vi "CleanUp.vi"(0 "object in":refnum<class "Valve.lvclass">, 5 "error in (no error)":errorcluster) -> (14 "object out":refnum<class "Valve.lvclass">, 19 "error out":errorcluster)   [LabVIEW 2019, in "Valve.lvclass"]
uses:
  Valve.lvclass
  Valve.lvclass/Valve.ctl
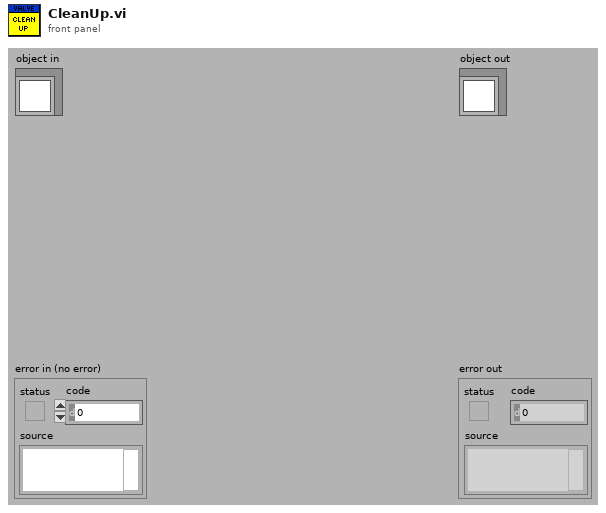
[diagram p1: front panel]
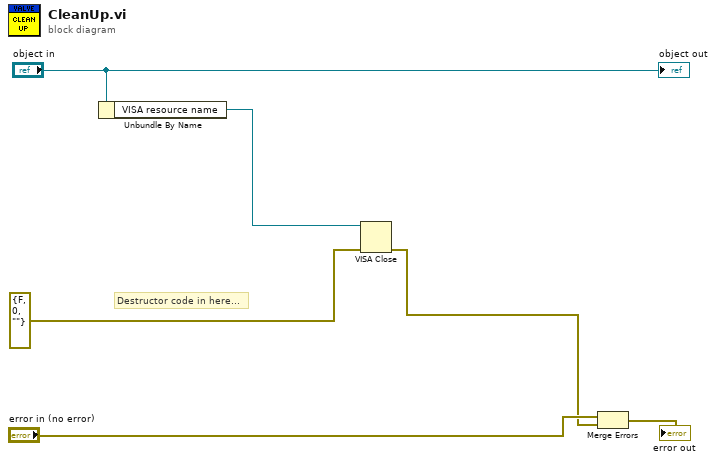
[diagram p0: block diagram]
diagram:
  # "Destructor code in here..."
  n1 = Unbundle By Name("object in") -> ("VISA resource name"=w1:refnum<visa-resource-name>)
  n2 = VISA Close(VISA resource name=w1, error in (no error)=errorcluster {"status"=FALSE, "code"=0, "source"=""}) -> (error out=w3:errorcluster)
  n3 = Merge Errors("error in (no error)", w3) -> (→"error out":errorcluster)
  "object out" <- "object in"
